vi "USB6343_Control_v1.5.vi"   [LabVIEW 2013]
uses:
  <vilib>/DAQmx/read.llb/DAQmx Read (Digital 1D Bool NChan 1Samp 1Line).vi
  <vilib>/DAQmx/read.llb/DAQmx Read (Analog 1D DBL NChan 1Samp).vi
  <vilib>/DAQmx/read.llb/DAQmx Read (Counter DBL 1Chan 1Samp).vi
  <vilib>/DAQmx/write.llb/DAQmx Write (Digital 1D Bool NChan 1Samp 1Line).vi
  <vilib>/DAQmx/write.llb/DAQmx Write (Analog 1D DBL NChan 1Samp).vi
  resources.vi
  <vilib>/DAQmx/miscellaneous.llb/DAQmx Fill In Error Info.vi
  <vilib>/DAQmx/configure/timing.llb/DAQmx Timing (Implicit).vi
  offsets.vi
  user-event.vi
types:
  T1 = cluster{"AI Task":refnum<k21>, "AO Task":refnum<k21>, "DO Task":refnum<k21>, "DI Task":refnum<k21>, "PWM x":refnum<k21>, "PWM y":refnum<k21>, "counter x":refnum<k21>, "counter y":refnum<k21>}
  T2 = cluster{"source":string, "channel":i32, "old value":dbl, "new value":dbl, "on/off":bool}
  T3 = cluster{"cmd":string, "channel":i32, "value":dbl, "on/off":bool, "return value":refnum<vi>}
  T4 = cluster{"data":dbl, "data":dbl, "data":dbl, "data":dbl}
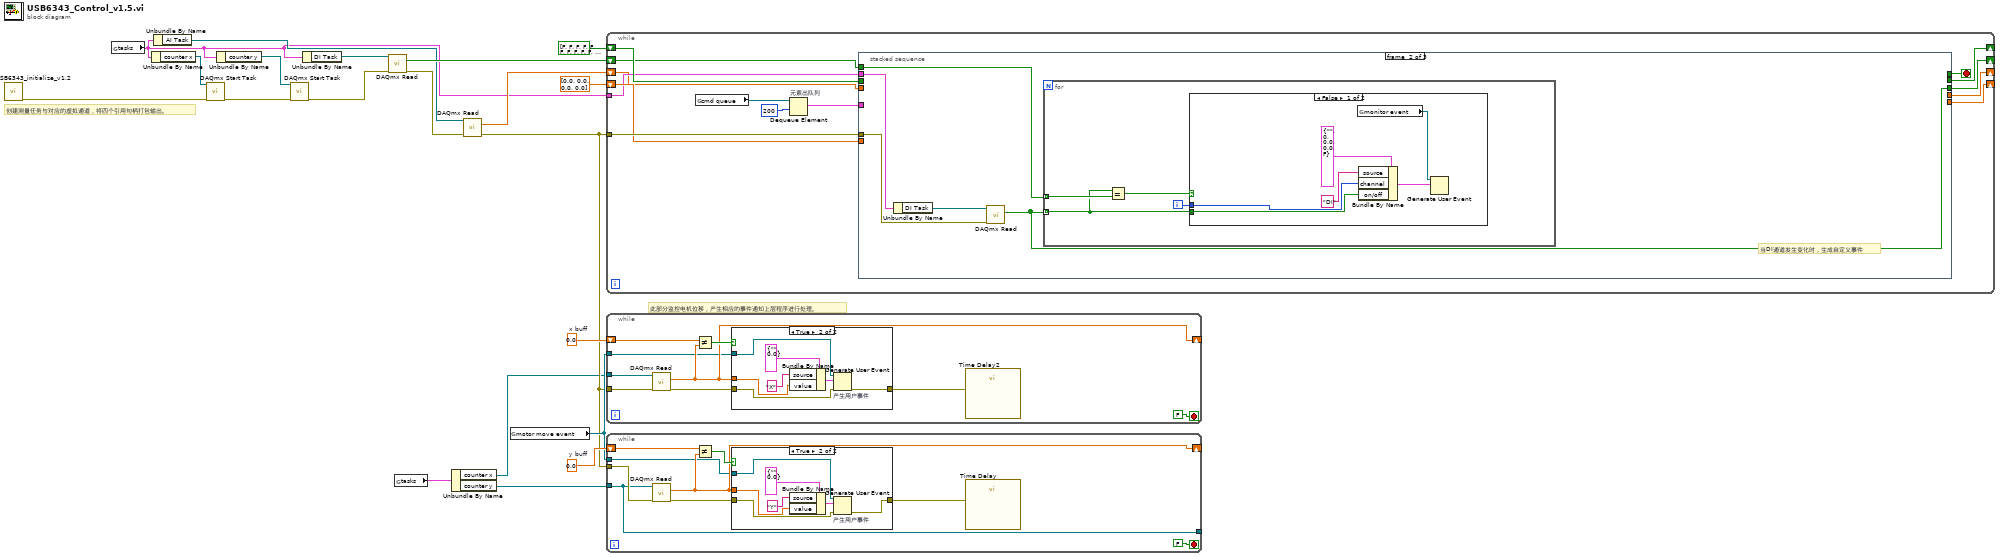
[diagram p0: block diagram]
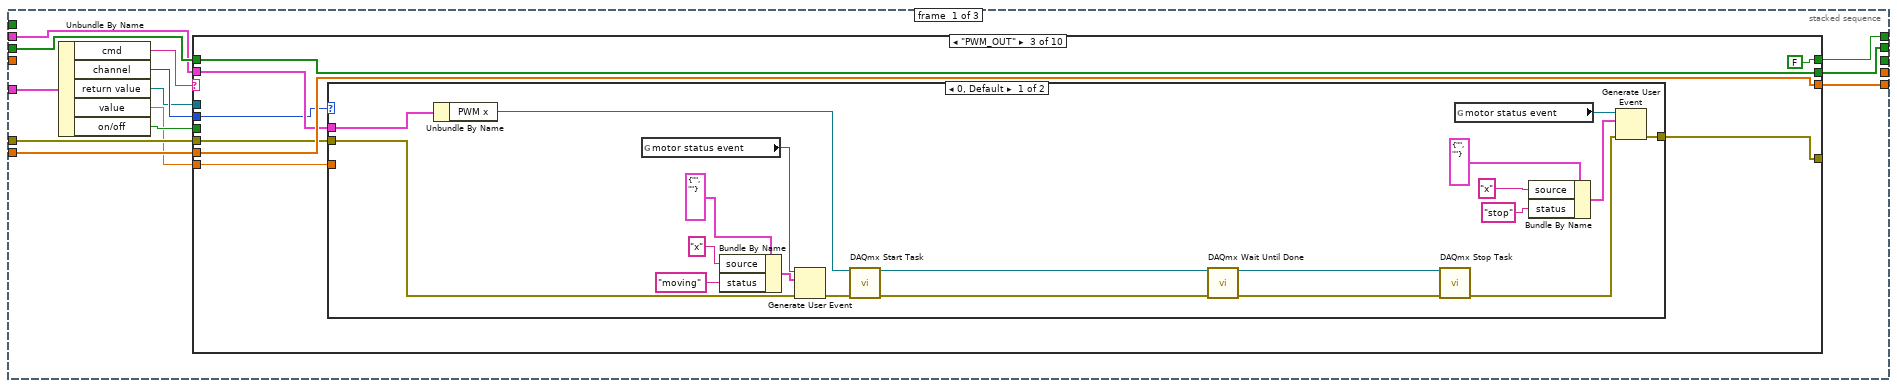
[diagram p4: hidden frame]
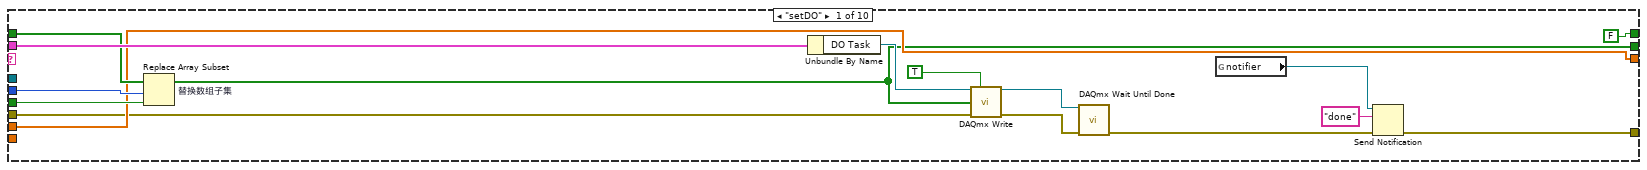
[diagram p5: hidden frame]
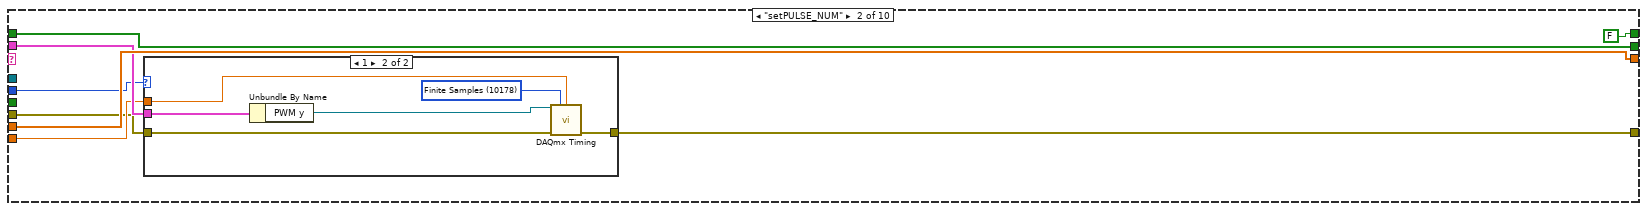
[diagram p6: hidden frame]
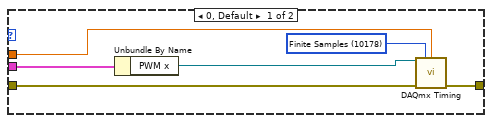
[diagram p7: hidden frame]
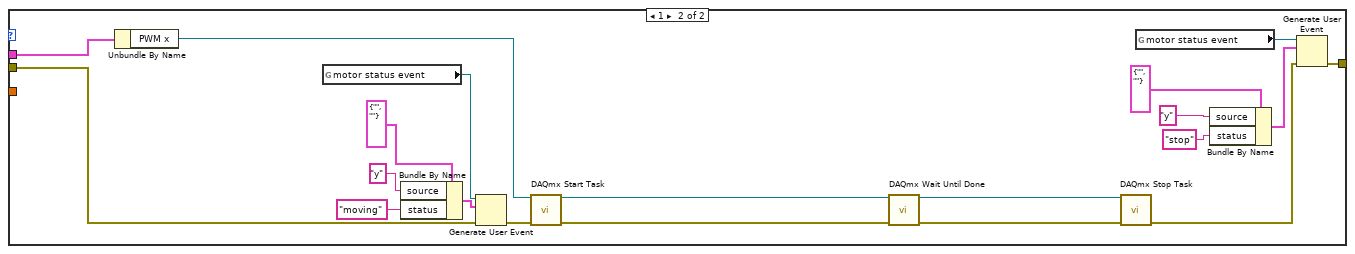
[diagram p8: hidden frame]
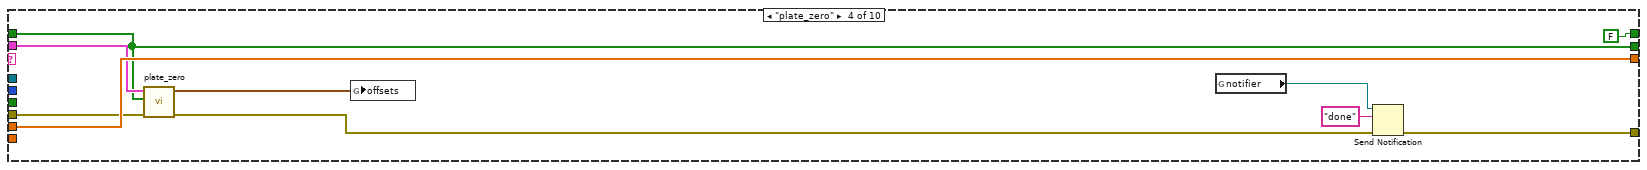
[diagram p9: hidden frame]
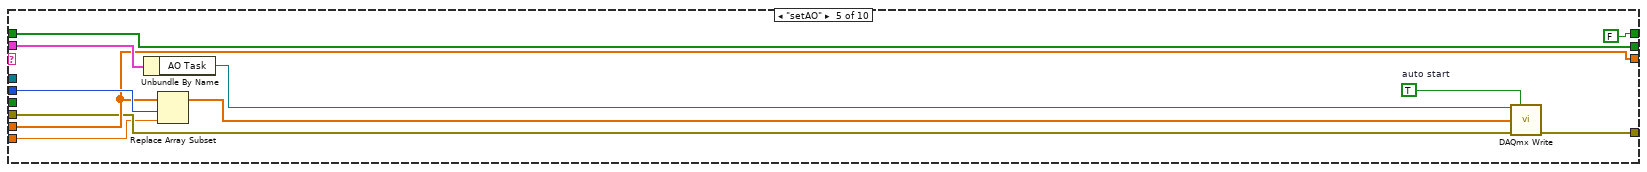
[diagram p10: hidden frame]
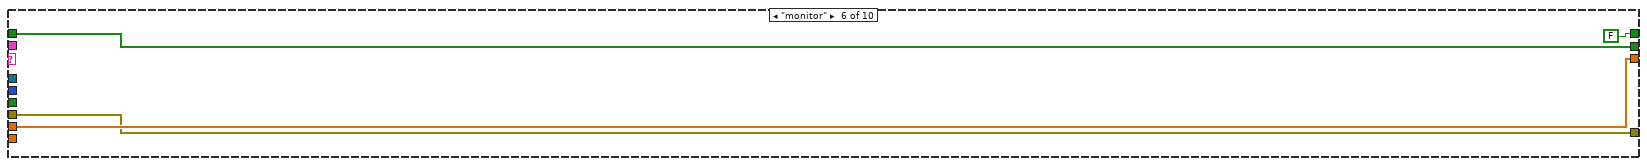
[diagram p11: hidden frame]
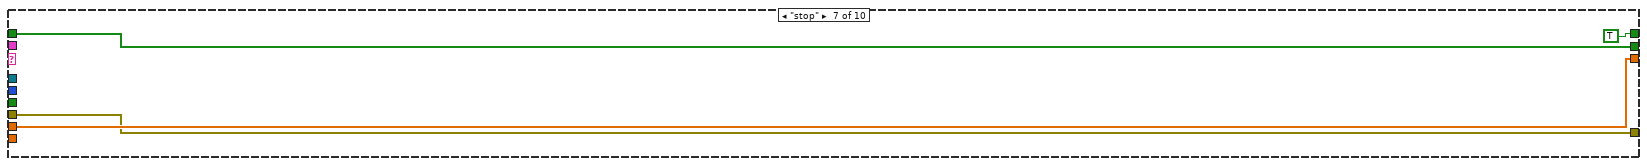
[diagram p12: hidden frame]
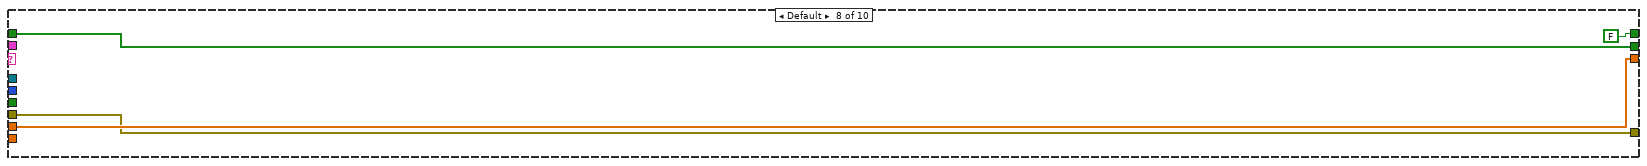
[diagram p13: hidden frame]
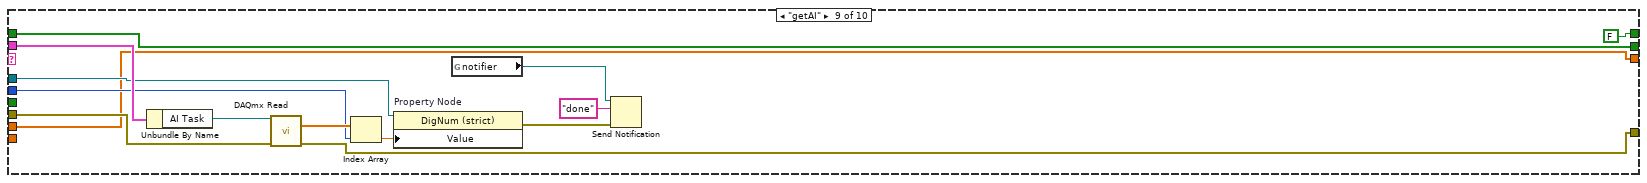
[diagram p14: hidden frame]
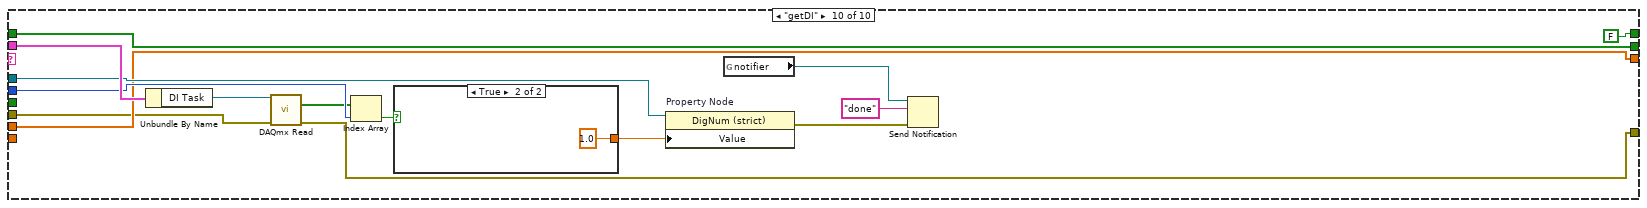
[diagram p15: hidden frame]
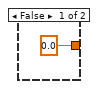
[diagram p16: hidden frame]
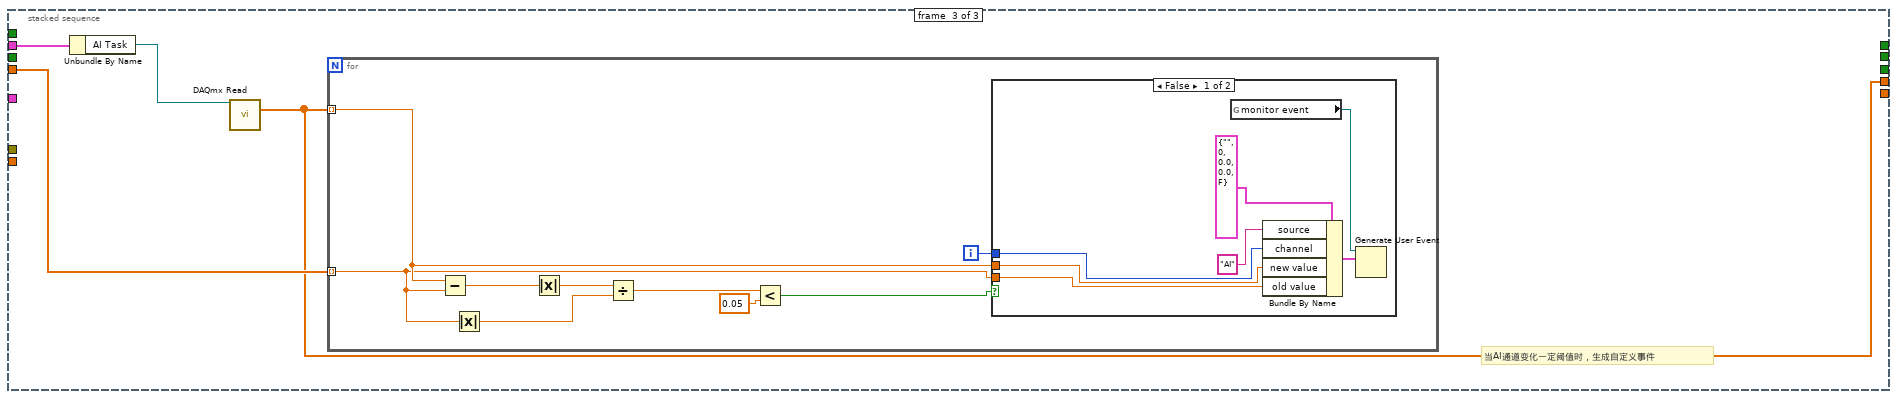
[diagram p18: hidden frame]
diagram:
  w6 = 0.0  # x buff
  w7 = 0.0  # y buff
  # "此部分监控电机位移，产生相应的事件通知上层程序进行处理。"
  # "创建测量任务与对应的虚拟通道，将四个引用句柄打包输出。"
  n1 = call "USB6343_initialize_v1.2.vi"() -> ("error out"=w9:errorcluster)  [unwired: 11 in]
  n2 = global read "resources.vi" "tasks"() -> (w8:T1)
  n3 = Unbundle By Name(w8) -> ("counter x"=w11:refnum<k21>)
  n4 = Unbundle By Name(w8) -> ("AI Task"=w15:refnum<k21>)
  n5 = call <vilib>:"DAQmx Start Task.vi"("task/channels in"=w11, "error in"=w9) -> ("error out"=w13:errorcluster)  [unwired: 12 in, 1 out]
  n6 = Unbundle By Name(w8) -> ("counter y"=w10:refnum<k21>)
  n7 = call <vilib>:"DAQmx Start Task.vi"("task/channels in"=w10, "error in"=w13) -> ("error out"=w12:errorcluster)  [unwired: 12 in, 1 out]
  n8 = Unbundle By Name(w8) -> ("DI Task"=w18:refnum<k21>)
  n9 = call-poly <vilib>:"DAQmx Read.vi"("task/channels in"=w18, "error in"=w12) -> ("data"=w17:bool[], "error out"=w16:errorcluster)  [unwired: 11 in, 1 out]
  n10 = global read "resources.vi" "tasks"() -> (w3:T1)
  n11 = Unbundle By Name(w3) -> ("counter x"=w2:refnum<k21>, "counter y"=w1:refnum<k21>)
  n12 = call-poly <vilib>:"DAQmx Read.vi"("task/channels in"=w15, "error in"=w16) -> ("data"=w14:dbl[], "error out"=w4:errorcluster)  [unwired: 11 in, 1 out]
  n13 = global read "resources.vi" "motor move event"() -> (w5:refnum<user-event>)
  n14 = while {
    tunnel: w8 -> [w28]
    tunnel: w4 -> [w34]
    shift-right: [w32] -> _
    shift-left: bool[] [FALSE, FALSE, FALSE, FALSE, FALSE, FALSE, FALSE, FALSE, FALSE, FALSE, FALSE, FALSE, FALSE, FALSE, FALSE, FALSE] -> [w33]
    shift-right: [w29] -> _
    shift-left: dbl[] [0.0, 0.0, 0.0, 0.0] ("data") -> [w30]
    shift-right: [w24] -> _
    shift-left: w17 -> [w25]
    shift-right: [w22] -> _
    shift-left: w14 -> [w23]
    stop <- w31 stop-if-true
    n15 = global read "resources.vi" "cmd queue"() -> (w21:refnum<queue>)
    n16 = Dequeue Element "元素出队列"(queue=w21, timeout in ms (-1)=200 ("超时毫秒(-1)")) -> (element=w27:T3)  [unwired: 1 in, 3 out]
    n17 = stacked-sequence {
      tunnel: w34 -> [w47 w198 _]
      tunnel: w33 -> [w46 _ _]
      tunnel: [w45 _ _] -> w32
      tunnel: [w44 _ _] -> w31
      tunnel: w30 -> [w43 _ _]
      tunnel: [w42 _ _] -> w29
      tunnel: w28 -> [w35 w200 w214]
      tunnel: w27 -> [w41 _ _]
      tunnel: w25 -> [_ w197 _]
      tunnel: [_ w196 _] -> w24
      tunnel: w23 -> [_ _ w212]
      tunnel: [_ _ w211] -> w22
      frame #0 {
        n18 = Unbundle By Name(w41) -> ("cmd"=w40:string, "channel"=w39:i32, "return value"=w38:refnum<vi>, "value"=w36:dbl, "on/off"=w37:bool)
        n19 = case shown="\"PWM_OUT\"" w40 {
          tunnel: w39 -> [w61 w65 w85 _ w150 _ _ _ w173 w191]
          tunnel: w35 -> [w63 w68 w88 w137 w152 _ _ _ w178 w193]
          tunnel: w47 -> [w55 w66 w86 w135 w144 w153 w157 w161 w175 w185]
          tunnel: w46 -> [w62 w69 w89 w136 w148 w156 w160 w164 w171 w190]
          tunnel: w37 -> [w60 _ _ _ _ _ _ _ _ _]
          tunnel: [w53 w69 w89 w136 w148 w156 w160 w164 w171 w190] -> w45
          tunnel: [FALSE FALSE FALSE FALSE FALSE FALSE TRUE FALSE FALSE FALSE] -> w44
          tunnel: w43 -> [w58 w70 w90 w140 w149 w155 w158 w162 w170 w189]
          tunnel: [w58 w70 w90 w140 w149 w155 w158 w162 w170 w189] -> w42
          tunnel: w38 -> [_ _ _ _ _ _ _ _ w176 w192]
          tunnel: [w57 w64 w84 w139 w142 w153 w157 w161 w168 w184] -> _
          tunnel: w36 -> [_ w67 w87 _ w143 _ _ _ _ _]
          frame "setDO" {
            n20 = Replace Array Subset "替换数组子集"(array=w62, new element=w60, index=w61) -> (w53:bool[])
            n21 = Unbundle By Name(w63) -> ("DO Task"=w54:refnum<k21>)
            n22 = call-poly <vilib>:"DAQmx Write.vi"("task/channels in"=w54, "auto start"=TRUE, "data"=w53, "error in"=w55) -> ("task out"=w49:refnum<k21>, "error out"=w51:errorcluster)  [unwired: 9 in, 1 out]
            n23 = call <vilib>:"DAQmx Wait Until Done.vi"("task/channels in"=w49, "error in"=w51) -> ("error out"=w50:errorcluster)  [unwired: 12 in, 1 out]
            n24 = global read "resources.vi" "notifier"() -> (w48:refnum<notifier>)
            n25 = Send Notification(notification="done" ("通知"), notifier=w48, error in (no error)=w50) -> (error out=w57:errorcluster)  [unwired: 1 out]
          }
          frame "setPULSE_NUM" {
            n26 = case shown="1" w65 {
              tunnel: w68 -> [w77 w83]
              tunnel: w67 -> [w74 w80]
              tunnel: w66 -> [w73 w79]
              tunnel: [w72 w78] -> w64
              frame 0, Default {
                w75 = 10178 items=["Finite Samples"=10178, "Continuous Samples"=10123, "Hardware Timed Single Point"=12522] ("sample mode")
                n27 = Unbundle By Name(w77) -> ("PWM x"=w76:refnum<k21>)
                n28 = call-poly <vilib>:"DAQmx Timing.vi"("task/channels in"=w76, "sample mode"=w75, "samples per channel"=w74, "error in"=w73) -> ("error out"=w72:errorcluster)  [unwired: 10 in, 1 out]
              }
              frame 1 {
                w81 = 10178 items=["Finite Samples"=10178, "Continuous Samples"=10123, "Hardware Timed Single Point"=12522] ("sample mode")
                n29 = Unbundle By Name(w83) -> ("PWM y"=w82:refnum<k21>)
                n30 = call-poly <vilib>:"DAQmx Timing.vi"("task/channels in"=w82, "sample mode"=w81, "samples per channel"=w80, "error in"=w79) -> ("error out"=w78:errorcluster)  [unwired: 10 in, 1 out]
              }
            }
          }
          frame "PWM_OUT" {
            n31 = case shown="0, Default" w85 {
              tunnel: w88 -> [w111 w131]
              tunnel: w87 -> [_ _]
              tunnel: w86 -> [w101 w122]
              tunnel: [w92 w114] -> w84
              frame 0, Default {
                n32 = Unbundle By Name(w111) -> ("PWM x"=w110:refnum<k21>)
                n33 = global read "resources.vi" "motor status event"() -> (w105:refnum<user-event>)
                n34 = Bundle By Name(cluster=cluster{"source":string, " status":string} {"source"="", " status"=""} ("event data"), "source"="x", "status"="moving") -> (w99:cluster{"source":string, " status":string})
                n35 = Generate User Event(user event=w105, event data cluster=w99, error in=w101) -> (error out=w100:errorcluster)  [unwired: 1 in, 1 out]
                n36 = call <vilib>:"DAQmx Start Task.vi"("task/channels in"=w110, "error in"=w100) -> ("task out"=w108:refnum<k21>, "error out"=w109:errorcluster)  [unwired: 12 in]
                n37 = call <vilib>:"DAQmx Wait Until Done.vi"("task/channels in"=w108, "error in"=w109) -> ("task out"=w106:refnum<k21>, "error out"=w107:errorcluster)  [unwired: 12 in]
                n38 = call <vilib>:"DAQmx Stop Task.vi"("task/channels in"=w106, "error in"=w107) -> ("error out"=w93:errorcluster)  [unwired: 12 in, 1 out]
                n39 = global read "resources.vi" "motor status event"() -> (w98:refnum<user-event>)
                n40 = Bundle By Name(cluster=cluster{"source":string, " status":string} {"source"="", " status"=""} ("event data"), "source"="x", "status"="stop") -> (w94:cluster{"source":string, " status":string})
                n41 = Generate User Event(user event=w98, event data cluster=w94, error in=w93) -> (error out=w92:errorcluster)  [unwired: 1 in, 1 out]
              }
              frame 1 {
                n42 = Unbundle By Name(w131) -> ("PWM x"=w130:refnum<k21>)
                n43 = global read "resources.vi" "motor status event"() -> (w125:refnum<user-event>)
                n44 = Bundle By Name(cluster=cluster{"source":string, " status":string} {"source"="", " status"=""} ("event data"), "source"="y", "status"="moving") -> (w113:cluster{"source":string, " status":string})
                n45 = Generate User Event(user event=w125, event data cluster=w113, error in=w122) -> (error out=w121:errorcluster)  [unwired: 1 in, 1 out]
                n46 = call <vilib>:"DAQmx Start Task.vi"("task/channels in"=w130, "error in"=w121) -> ("task out"=w128:refnum<k21>, "error out"=w129:errorcluster)  [unwired: 12 in]
                n47 = call <vilib>:"DAQmx Wait Until Done.vi"("task/channels in"=w128, "error in"=w129) -> ("task out"=w126:refnum<k21>, "error out"=w127:errorcluster)  [unwired: 12 in]
                n48 = call <vilib>:"DAQmx Stop Task.vi"("task/channels in"=w126, "error in"=w127) -> ("error out"=w115:errorcluster)  [unwired: 12 in, 1 out]
                n49 = global read "resources.vi" "motor status event"() -> (w120:refnum<user-event>)
                n50 = Bundle By Name(cluster=cluster{"source":string, " status":string} {"source"="", " status"=""} ("event data"), "source"="y", "status"="stop") -> (w116:cluster{"source":string, " status":string})
                n51 = Generate User Event(user event=w120, event data cluster=w116, error in=w115) -> (error out=w114:errorcluster)  [unwired: 1 in, 1 out]
              }
            }
          }
          frame "plate_zero" {
            n52 = call "plate_zero.vi"("error in"=w135, "DO array"=w136, "tasks"=w137) -> ("error out"=w134:errorcluster, "offsets"=w133:T4)  [unwired: 7 in]
            n53 = global write "offsets.vi" "offsets"(w133) -> ()
            n54 = global read "resources.vi" "notifier"() -> (w132:refnum<notifier>)
            n55 = Send Notification(notification="done", notifier=w132, error in (no error)=w134) -> (error out=w139:errorcluster)  [unwired: 1 out]
          }
          frame "setAO" {
            w146 = TRUE  # auto start
            n56 = Unbundle By Name(w152) -> ("AO Task"=w151:refnum<k21>)
            n57 = Replace Array Subset(array=w149, new element=w143, index=w150) -> (w147:dbl[])
            n58 = call-poly <vilib>:"DAQmx Write.vi"("task/channels in"=w151, "auto start"=w146, "data"=w147, "error in"=w144) -> ("error out"=w142:errorcluster)  [unwired: 9 in, 2 out]
          }
          frame "monitor" {
          }
          frame "stop" {
          }
          frame Default {
          }
          frame "getAI" {
            n59 = Unbundle By Name(w178) -> ("AI Task"=w177:refnum<k21>)
            n60 = call-poly <vilib>:"DAQmx Read.vi"("task/channels in"=w177, "error in"=w175) -> ("data"=w174:dbl[], "error out"=w168:errorcluster)  [unwired: 11 in, 1 out]
            n61 = Index Array(array=w174, index=w173) -> (element=w172:dbl)
            n62 = property on="Property Node" class="DigNum (strict)"(reference=w176, "Value"=w172) -> (error out=w166:errorcluster)  [unwired: 1 in, 1 out]
            n63 = global read "resources.vi" "notifier"() -> (w165:refnum<notifier>)
            n64 = Send Notification(notification="done" ("通知"), notifier=w165, error in (no error)=w166) -> ()  [unwired: 2 out]
          }
          frame "getDI" {
            n65 = Unbundle By Name(w193) -> ("DI Task"=w183:refnum<k21>)
            n66 = call-poly <vilib>:"DAQmx Read.vi"("task/channels in"=w183, "error in"=w185) -> ("data"=w182:bool[], "error out"=w184:errorcluster)  [unwired: 11 in, 1 out]
            n67 = Index Array(array=w182, index=w191) -> (element=w181:bool)
            n68 = case shown="True" w181 {
              tunnel: [0.0 1.0] -> w180
              frame False {
              }
              frame True {
              }
            }
            n69 = property on="Property Node" class="DigNum (strict)"(reference=w192, "Value"=w180) -> (error out=w186:errorcluster)  [unwired: 1 in, 1 out]
            n70 = global read "resources.vi" "notifier"() -> (w179:refnum<notifier>)
            n71 = Send Notification(notification="done" ("通知"), notifier=w179, error in (no error)=w186) -> ()  [unwired: 2 out]
          }
        }
      }
      frame #1 {
        # "当DI通道发生变化时，生成自定义事件"
        n72 = Unbundle By Name(w200) -> ("DI Task"=w199:refnum<k21>)
        n73 = call-poly <vilib>:"DAQmx Read.vi"("task/channels in"=w199, "error in"=w198) -> ("data"=w196:bool[])  [unwired: 11 in, 2 out]
        n74 = for {
          tunnel: w196 -> [w201] mode=indexing
          tunnel: w197 -> [w204] mode=indexing
          i -> [w202]
          n75 = Equal?(x=w201, y=w204) -> (x = y?=w203:bool)
          n76 = case shown="False" w203 {
            tunnel: w202 -> [w208 _]
            tunnel: w201 -> [w207 _]
            frame False {
              n77 = global read "user-event.vi" "monitor event"() -> (w205:refnum<user-event>)
              n78 = Bundle By Name(cluster=T2 {"source"="", "channel"=0, "old value"=0.0, "new value"=0.0, "on/off"=FALSE} ("事件数据"), "source"="DI", "channel"=w208, "on/off"=w207) -> (w206:T2)
              n79 = Generate User Event(user event=w205, event data cluster=w206) -> ()  [unwired: 2 in, 2 out]
            }
            frame True {
            }
          }
        }
      }
      frame #2 {
        # "当AI通道变化一定阈值时，生成自定义事件"
        n80 = Unbundle By Name(w214) -> ("AI Task"=w213:refnum<k21>)
        n81 = call-poly <vilib>:"DAQmx Read.vi"("task/channels in"=w213) -> ("data"=w211:dbl[])  [unwired: 12 in, 2 out]
        n82 = for {
          tunnel: w211 -> [w216] mode=indexing
          tunnel: w212 -> [w215] mode=indexing
          i -> [w217]
          n83 = Subtract(x=w216, y=w215) -> (x-y=w223:dbl)
          n84 = Absolute Value(x=w215) -> (abs(x)=w221:dbl)
          n85 = Absolute Value(x=w223) -> (abs(x)=w222:dbl)
          n86 = Divide(x=w222, y=w221) -> (x/y=w220:dbl)
          n87 = Less?(x=w220, y=0.05) -> (x < y?=w218:bool)
          n88 = case shown="False" w218 {
            tunnel: w217 -> [w228 _]
            tunnel: w216 -> [w227 _]
            tunnel: w215 -> [w226 _]
            frame False {
              n89 = global read "user-event.vi" "monitor event"() -> (w224:refnum<user-event>)
              n90 = Bundle By Name(cluster=T2 {"source"="", "channel"=0, "old value"=0.0, "new value"=0.0, "on/off"=FALSE} ("事件数据"), "source"="AI", "channel"=w228, "new value"=w227, "old value"=w226) -> (w225:T2)
              n91 = Generate User Event(user event=w224, event data cluster=w225) -> ()  [unwired: 2 in, 2 out]
            }
            frame True {
            }
          }
        }
      }
    }
  }
  n92 = while {
    tunnel: w2 -> [w237]
    tunnel: w4 -> [w239]
    shift-right: [w235] -> _
    shift-left: w6 -> [w238]
    tunnel: w5 -> [w231]
    stop <- FALSE stop-if-true
    n93 = call-poly <vilib>:"DAQmx Read.vi"("task/channels in"=w237, "error in"=w239) -> ("data"=w235:dbl, "error out"=w234:errorcluster)  [unwired: 11 in, 1 out]
    n94 = Not Equal?(x=w238, y=w235) -> (x != y?=w236:bool)
    n95 = case shown="True" w236 {
      tunnel: w235 -> [_ w241]
      tunnel: w234 -> [w240 w244]
      tunnel: [w240 w243] -> w232
      tunnel: w231 -> [_ w242]
      frame False {
      }
      frame True {
        n96 = Bundle By Name(cluster=cluster{"source":string, "value":dbl} {"source"="", "value"=0.0} ("事件数据"), "source"="X", "value"=w241) -> (w245:cluster{"source":string, "value":dbl})
        n97 = Generate User Event "产生用户事件"(user event=w242, event data cluster=w245, error in=w244) -> (error out=w243:errorcluster)  [unwired: 1 in, 1 out]
      }
    }
    n98 = call "Time Delay2"("error in (no error)"=w232) -> ()  [unwired: 10 in, 1 out]
  }
  n99 = while {
    tunnel: [w248] -> _
    tunnel: w4 -> [w256]
    shift-right: [w253] -> _
    shift-left: w7 -> [w255]
    tunnel: w5 -> [w249]
    tunnel: w1 -> [w248]
    stop <- FALSE stop-if-true
    n100 = call-poly <vilib>:"DAQmx Read.vi"("task/channels in"=w248, "error in"=w256) -> ("data"=w253:dbl, "error out"=w252:errorcluster)  [unwired: 11 in, 1 out]
    n101 = Not Equal?(x=w255, y=w253) -> (x != y?=w254:bool)
    n102 = case shown="True" w254 {
      tunnel: w253 -> [_ w258]
      tunnel: w252 -> [w257 w260]
      tunnel: [w257 w259] -> w250
      tunnel: w249 -> [_ w261]
      frame False {
      }
      frame True {
        n103 = Bundle By Name(cluster=cluster{"source":string, "value":dbl} {"source"="", "value"=0.0} ("事件数据"), "source"="Y", "value"=w258) -> (w262:cluster{"source":string, "value":dbl})
        n104 = Generate User Event "产生用户事件"(user event=w261, event data cluster=w262, error in=w260) -> (error out=w259:errorcluster)  [unwired: 1 in, 1 out]
      }
    }
    n105 = call "Time Delay"("error in (no error)"=w250) -> ()  [unwired: 10 in, 1 out]
  }
